vi "Post-Build Custom Action - Synchronize Palette with Directory.vi"(10 "Variant":variant) -> (0 "error out":errorcluster)   [LabVIEW 2015]
uses:
  <vilib>/Palette API/Palette Menu/Public Type Define/Palette type.ctl
  <vilib>/Palette API/Palette Menu/Palette Menu.lvlib
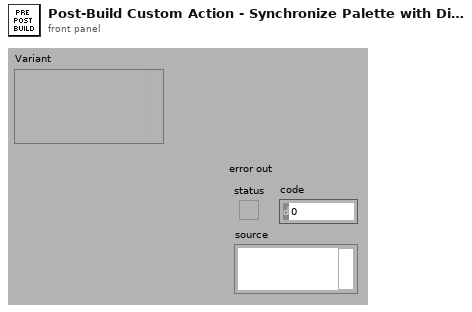
[diagram p1: front panel]
types:
  T1 = typedef "Palette Menu.lvlib/Palette type.ctl" = i32
  T2 = typedef "Palette Menu.lvlib/Palette Data.ctl" = cluster{"display name":string, "view format":T3, "palette width":i16, "items":T4, "256 color icon":picture, "B&W color icon":picture, "help information":T6, "palette description":string, "synchronize information":T7}
  T3 = typedef "Palette Menu.lvlib/View Format.ctl" = u16
  T4 = typedef "Palette Menu.lvlib/Items.ctl" = T5[]
  T5 = typedef "Palette Menu.lvlib/Item.ctl" = cluster{"item path":path, "library path (.lvlib)":path, "use default lvlib palette":bool, "short name":string, "place VI contents":bool, "hide synchronized item":bool, "reserve spot for synch item":bool, "configure when placing VI contents":bool}
  T6 = typedef "Palette Menu.lvlib/Help Info.ctl" = cluster{"help tag":string, "help file path ":path}
  T7 = typedef "Palette Menu.lvlib/Synchronize Info.ctl" = cluster{"synchronize with directory":bool, "synchronize directory path":path}
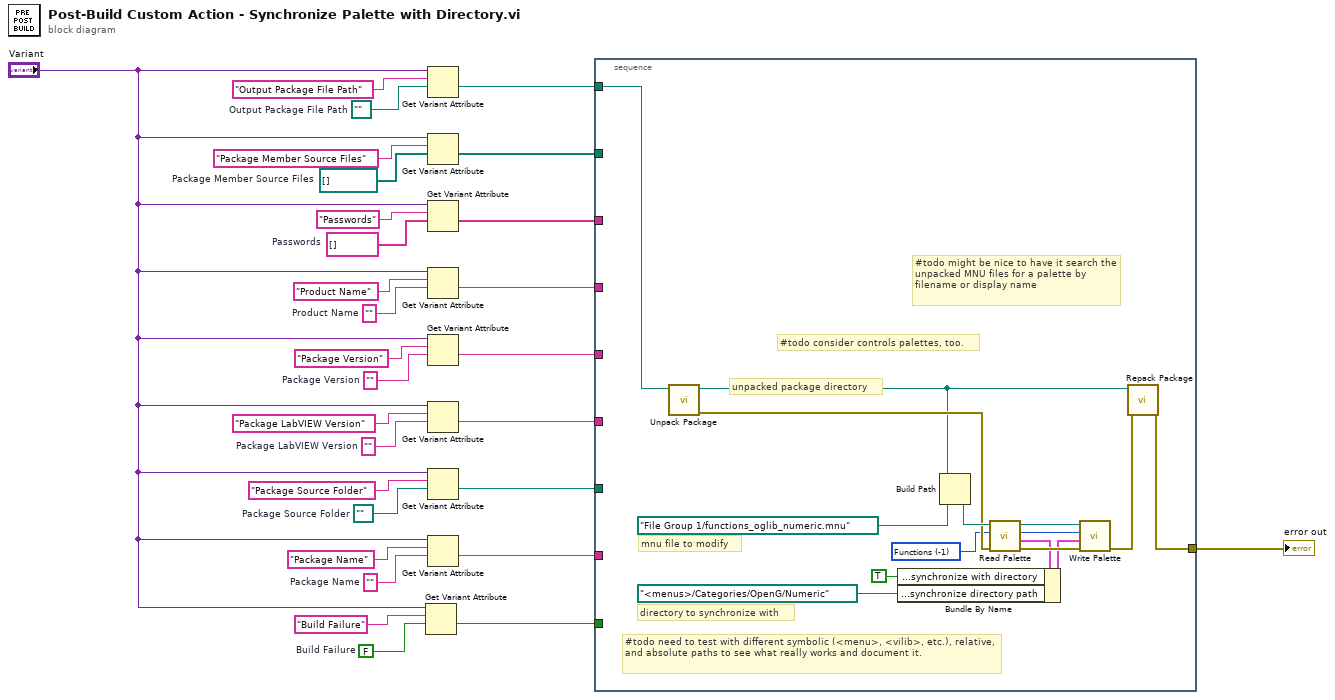
[diagram p0: block diagram]
diagram:
  w4 = FALSE  # Build Failure
  w14 = path ""  # Package Source Folder
  w15 = ""  # Package Name
  w18 = ""  # Package LabVIEW Version
  w20 = ""  # Package Version
  w22 = ""  # Product Name
  w24 = string[] []  # Passwords
  w26 = path[] []  # Package Member Source Files
  w28 = path ""  # Output Package File Path
  n1 = Get Variant Attribute(Variant="Variant", name="Build Failure", default value (empty Variant)=w4) -> (value=w2:bool)  [unwired: 1 in, 3 out]
  n2 = Get Variant Attribute(Variant="Variant", name="Output Package File Path", default value (empty Variant)=w28) -> (value=w13:path)  [unwired: 1 in, 3 out]
  n3 = Get Variant Attribute(Variant="Variant", name="Package Member Source Files", default value (empty Variant)=w26) -> (value=w12:path[])  [unwired: 1 in, 3 out]
  n4 = Get Variant Attribute(Variant="Variant", name="Passwords", default value (empty Variant)=w24) -> (value=w11:string[])  [unwired: 1 in, 3 out]
  n5 = Get Variant Attribute(Variant="Variant", name="Product Name", default value (empty Variant)=w22) -> (value=w10:string)  [unwired: 1 in, 3 out]
  n6 = Get Variant Attribute(Variant="Variant", name="Package Version", default value (empty Variant)=w20) -> (value=w9:string)  [unwired: 1 in, 3 out]
  n7 = Get Variant Attribute(Variant="Variant", name="Package LabVIEW Version", default value (empty Variant)=w18) -> (value=w8:string)  [unwired: 1 in, 3 out]
  n8 = Get Variant Attribute(Variant="Variant", name="Package Source Folder", default value (empty Variant)=w14) -> (value=w7:path)  [unwired: 1 in, 3 out]
  n9 = Get Variant Attribute(Variant="Variant", name="Package Name", default value (empty Variant)=w15) -> (value=w6:string)  [unwired: 1 in, 3 out]
  n10 = stacked-sequence {
    tunnel: w13 -> [w43]
    tunnel: w12 -> [_]
    tunnel: w11 -> [_]
    tunnel: w10 -> [_]
    tunnel: w9 -> [_]
    tunnel: w8 -> [_]
    tunnel: w7 -> [_]
    tunnel: w6 -> [_]
    tunnel: w2 -> [_]
    tunnel: [w33] -> w1
    frame #0 {
      w30 = T1 -1 items=["Functions"=-1, "Controls"=-2] ("palette type")
      # "#todo need to test with different symbolic (<menu>, <vilib>, etc.), relative, and absolute paths to see what really works and document it."
      # "#todo consider controls palettes, too."
      # "unpacked package directory"
      # "directory to synchronize with"
      # "mnu file to modify"
      # "#todo might be nice to have it search the unpacked MNU files for a palette by filename or display name"
      n11 = call "Unpack Package.vi"("Package File"=w43) -> ("error out"=w32:errorcluster, "Unpacked Package Directory"=w31:path)  [unwired: 8 in, 1 out]
      n12 = Build Path(base path=w31, name or relative path=path "File Group 1/functions_oglib_numeric.mnu" ("Unpacked File")) -> (appended path=w42:path)
      n13 = call <vilib>:"Read Palette.vi"("error in (no error)"=w32, "palette type"=w30, "palette path"=w42) -> ("error out"=w40:errorcluster, "palette data"=w37:T2, "duplicate palette path"=w36:path)  [unwired: 6 in]
      n14 = Bundle By Name(cluster=w37, "synchronize information.synchronize with directory"=TRUE, "synchronize information.synchronize directory path"=path "<menus>/Categories/OpenG/Numeric" ("Unpacked File")) -> (w38:T2)
      n15 = call <vilib>:"Write Palette.vi"("error in (no error)"=w40, "palette data"=w38, "palette type"=w30, "palette path"=w36) -> ("error out"=w34:errorcluster)  [unwired: 7 in]
      n16 = call "Repack Package.vi"("error in (no error)"=w34, "Directory to repack"=w31) -> ("error out"=w33:errorcluster)  [unwired: 9 in]
    }
  }
  "error out" <- w1
